vi "LABVIEW FINGERS.vi"() -> ()   [LabVIEW 2017]
uses:
  <vilib>/Instr/_visa.llb/VISA Configure Serial Port (Instr).vi
  <vilib>/Utility/file.llb/Write Delimited Spreadsheet (I64).vi
panel:
  out "new file path (Not A Path if cancelled)":path
  in  "name or relative path":string="C:\\FingerTests"
  out "appended path":path
  in  "Save":bool
  out "x-y":u32
  out "fps":dbl
  in  "Serial Settings:Number of Bytes at Serial Port":u32=16
  out "Waveform Chart":i32(graph)
  out "return count":u32
  in  "flow control (0:none)":u16(ring) items=["None", "XON/XOFF", "RTS/CTS", "XON/XOFF & RTS/CTS", "DTR/DSR", "XON/XOFF & DTR/DSR"]
  in  "stop bits (10: 1 bit)":u16(ring)=10 items=["1.0"=10, "1.5"=15, "2.0"=20]
  in  "error in (no error)":errorcluster
  in  "parity (0:none)":enum16{"None", "Odd", "Even", "Mark", "Space"}(ring)
  in  "data bits (8)":u16=8 min=5 max=8 step=1
  in  "baud rate (9600)":u32=9600
  out "read buffer":string
  in  "stop":bool
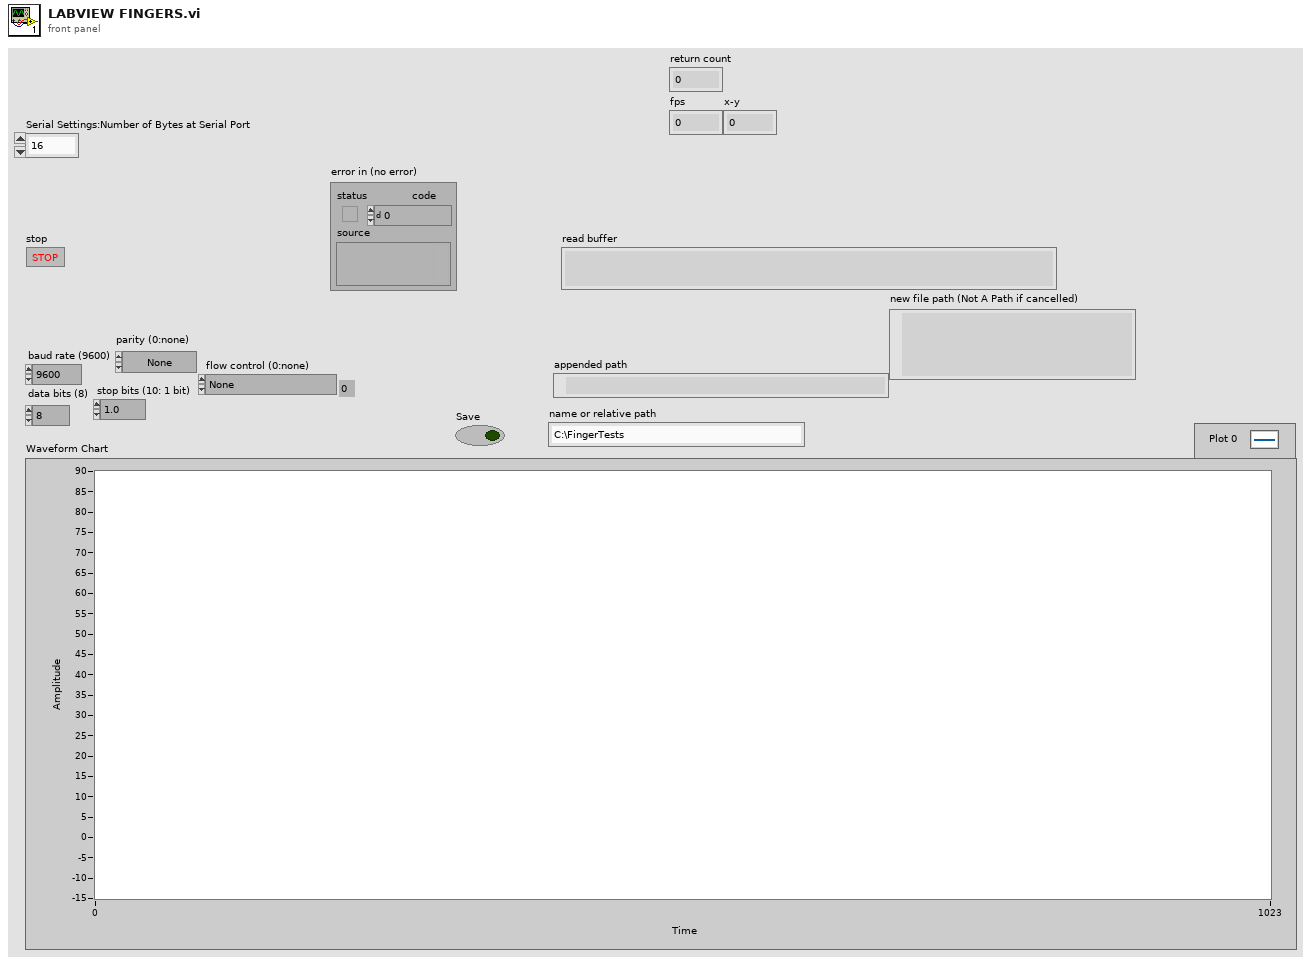
[diagram p1: front panel]
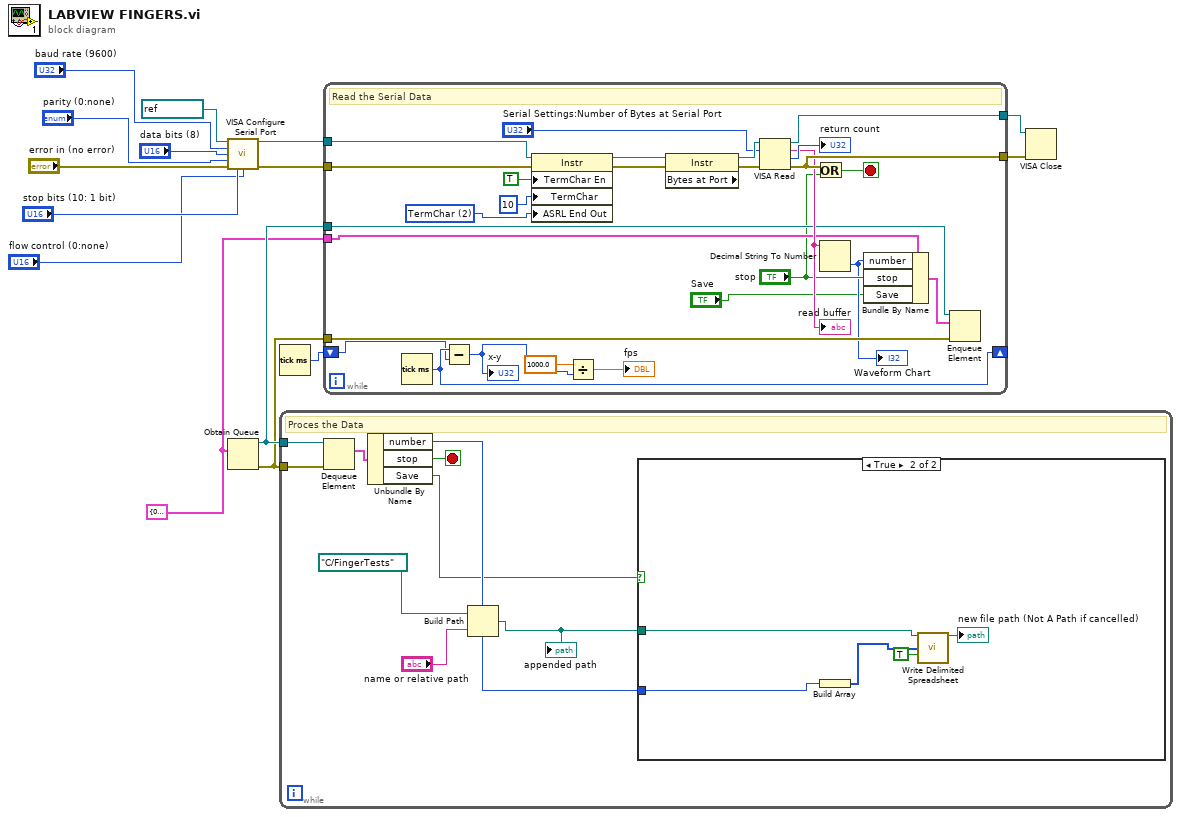
[diagram p0: block diagram]
diagram:
  w2 = cluster{"number":i32, "stop":bool, "Save":bool} {"number"=0, "stop"=FALSE, "Save"=FALSE}
  n1 = call-poly "VISA Configure Serial Port"("VISA resource name"=refnum<visa-resource-name> "COM4", "baud rate (9600)"="baud rate (9600)", "data bits (8)"="data bits (8)", "parity (0:none)"="parity (0:none)", "error in (no error)"="error in (no error)", "stop bits (10: 1 bit)"="stop bits (10: 1 bit)", "flow control (0:none)"="flow control (0:none)") -> ("VISA resource name out"=w6:refnum<visa-resource-name>, "error out"=w5:errorcluster)  [unwired: 7 in]
  n2 = Obtain Queue(element data type=w2) -> (queue out=w4:refnum<queue>, error out=w3:errorcluster)  [unwired: 4 in, 1 out]
  n3 = Tick Count (ms)() -> (millisecond timer value=w1:u32)
  n4 = while {
    tunnel: w4 -> [w24]
    tunnel: w3 -> [w23]
    stop <- w21 stop-if-true
    # "Proces the Data"
    n5 = Dequeue Element(queue=w24, error in (no error)=w23) -> (element=w22:cluster{"number":i32, "stop":bool, "Save":bool})  [unwired: 1 in, 3 out]
    n6 = Unbundle By Name(w22) -> ("number"=w17:i32, "stop"=w21:bool, "Save"=w16:bool)
    n7 = Build Path(base path=path "C:/FingerTests" ("Filename"), name or relative path="name or relative path") -> (appended path=w18:path)
    "appended path" <- w18
    n8 = case shown="True" w16 {
      tunnel: w17 -> [_ w28]
      tunnel: w18 -> [_ w29]
      frame False {
      }
      frame True {
        n9 = Build Array(w28) -> (w27:i32[])
        n10 = call-poly <vilib>:"Write Delimited Spreadsheet.vi"("file path (dialog if empty)"=w29, "1D data"=w27, "append to file? (new file:F)"=TRUE) -> ("new file path (Not A Path if cancelled)"=→"new file path (Not A Path if cancelled)":path)  [unwired: 11 in, 1 out]
      }
    }
  }
  n11 = while {
    tunnel: [w52] -> w7
    tunnel: [w54] -> w8
    tunnel: w6 -> [w51]
    tunnel: w5 -> [w50]
    tunnel: w4 -> [w41]
    tunnel: w3 -> [w40]
    tunnel: w2 -> [w39]
    shift-right: [w35] -> _
    shift-left: w1 -> [w34]
    stop <- w53 stop-if-true
    w47 = u16 2 items=["None", "Last Bit", "TermChar", "Break"] ("Serial Settings:End Mode for Writes")
    # "Read the Serial Data"
    n12 = Tick Count (ms)() -> (millisecond timer value=w35:u32)
    n13 = Subtract(x=w35, y=w34) -> (x-y=w33:u32)
    "x-y" <- w33
    n14 = property class="Instr"(reference=w51, error in=w50, "TermChar En"=TRUE ("Message Based Settings:Termination Character Enable"), "TermChar"=u8 10 ("Message Based Settings:Termination Character"), "ASRL End Out"=w47) -> (reference out=w46:refnum<visa-resource-name>, error out=w45:errorcluster)
    n15 = Divide(x=1000.0, y=w33) -> (x/y=→"fps":dbl)
    n16 = property class="Instr" props=["Bytes at Port"](reference=w46, error in=w45) -> (reference out=w56:refnum<visa-resource-name>, error out=w55:errorcluster)  [unwired: 1 out]
    n17 = VISA Read(VISA resource name=w56, byte count="Serial Settings:Number of Bytes at Serial Port", error in (no error)=w55) -> (VISA resource name out=w54:refnum<visa-resource-name>, read buffer=w43:string, return count=→"return count":u32, error out=w52:errorcluster)
    "read buffer" <- w43
    n18 = Or(x=w52, y="stop") -> (x .or. y?=w53:bool)
    n19 = Decimal String To Number(string=w43) -> (number=w31:i32)  [unwired: 2 in, 1 out]
    "Waveform Chart" <- w31
    n20 = Bundle By Name(cluster=w39, "number"=w31, "stop"="stop", "Save"="Save") -> (w37:cluster{"number":i32, "stop":bool, "Save":bool})
    n21 = Enqueue Element(queue=w41, element=w37, error in (no error)=w40) -> ()  [unwired: 1 in, 3 out]
  }
  n22 = VISA Close(VISA resource name=w8, error in (no error)=w7) -> ()  [unwired: 1 out]
